vi "Pot Single Line-UR6060.vi"() -> ()   [LabVIEW 2017]
uses:
  Shared Components/Config Manager Class/Type Definitions/Potting Parameters.ctl
  <vilib>/Utility/error.llb/DialogType.ctl
  Shared Components/Config Manager Class/Type Definitions/Camera Enum.ctl
  Shared Components/Gantry Class/Type Definitions/Init_Modes.ctl
  Shared Components/Gantry Class/Type Definitions/Virtual Modes.ctl
  Shared Components/Config Manager Class/Type Definitions/Potting Surface Type.ctl
  Shared Components/Gantry Class/Gantry Class.lvclass
  Shared Components/SyringeTool Class/SyringeTool Class.lvclass
  Shared Components/WorkTable Class/WorkTable Class.lvclass
  Shared Components/Vec3d Class/Vec3d Class.lvclass
panel:
  out "error out":errorcluster
  in  "Potting Parameters":T1={"Curing Param A"=0.0, "Curing Param B"=0.0, "Speed Nominal"=0.5, "Time Nominal"=2.0, "Turn-on Time"=0.5, "Turn-off Time"=0.1, "Safe Height Offset"=0.0, "Tip Height"=0.18, "Width of Line"=0.0, "Number of lines"=1.0, "Distance between lines"=0.1}
  out "Image":T2(plugin-control)
  in  "stop":bool
  in  "Config Folder":path=path "C:/Users/Husker/Desktop/gantry/Config"
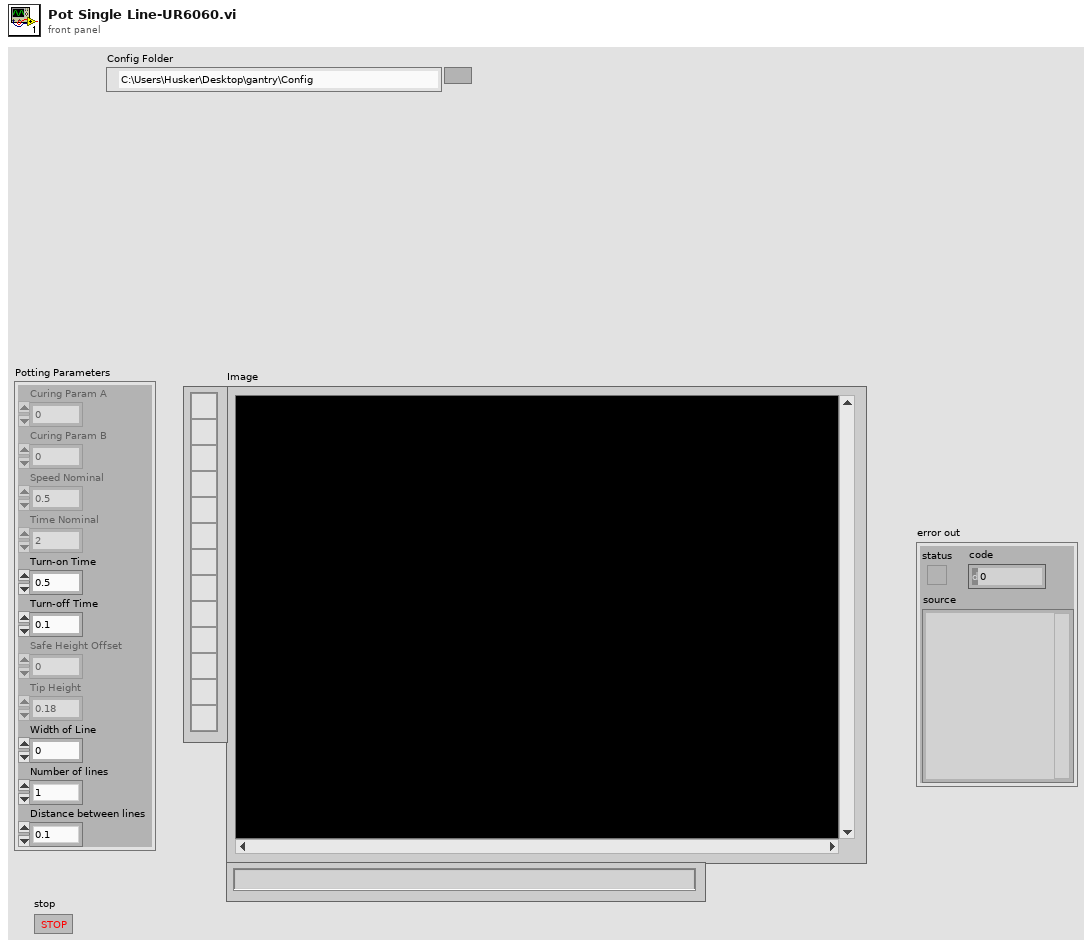
[diagram p1: front panel]
types:
  T1 = typedef "Potting Parameters.ctl" = cluster{"Curing Param A":dbl, "Curing Param B":dbl, "Speed Nominal":dbl, "Time Nominal":dbl, "Turn-on Time":dbl, "Turn-off Time":dbl, "Safe Height Offset":dbl, "Tip Height":dbl, "Width of Line":dbl, "Number of lines":dbl, "Distance between lines":dbl}
  T2 = typedef "IMAQ Image.ctl" = refnum<image>
  T3 = typedef "Virtual Modes.ctl" = enum16{"Nonvirtual", "Pseudovirtual", "Virtual"}
  T4 = typedef "Init_Modes.ctl" = enum16{"Full", "Robot Only", "Dispenser Only", "Cameras Only", "Robot and Cameras", "Robot and Cameras and Dispenser", "Manifold Only"}
  T5 = typedef "Camera Enum.ctl" = enum16{"GANTRY HEAD", "NEEDLE CALIBRATION X", "NEEDLE CALIBRATION Y", "STAND CAMERA", "SIMRAN WEBCAM"}
  T6 = typedef "DialogType.ctl" = u16
  T7 = typedef "Worktable_Syringe.ctl" = cluster{"Syringe Holder":enum16{"Empty", "Populated", "Calibrated"}, "Mixing Time":timestamp, "Tip Offset":refnum<class "Vec3d Class.lvclass">}
  T8 = typedef "Potting Surface Type.ctl" = enum16{"default", "hdi_edge_pads", "bbm_edge_pads", "address_pads"}
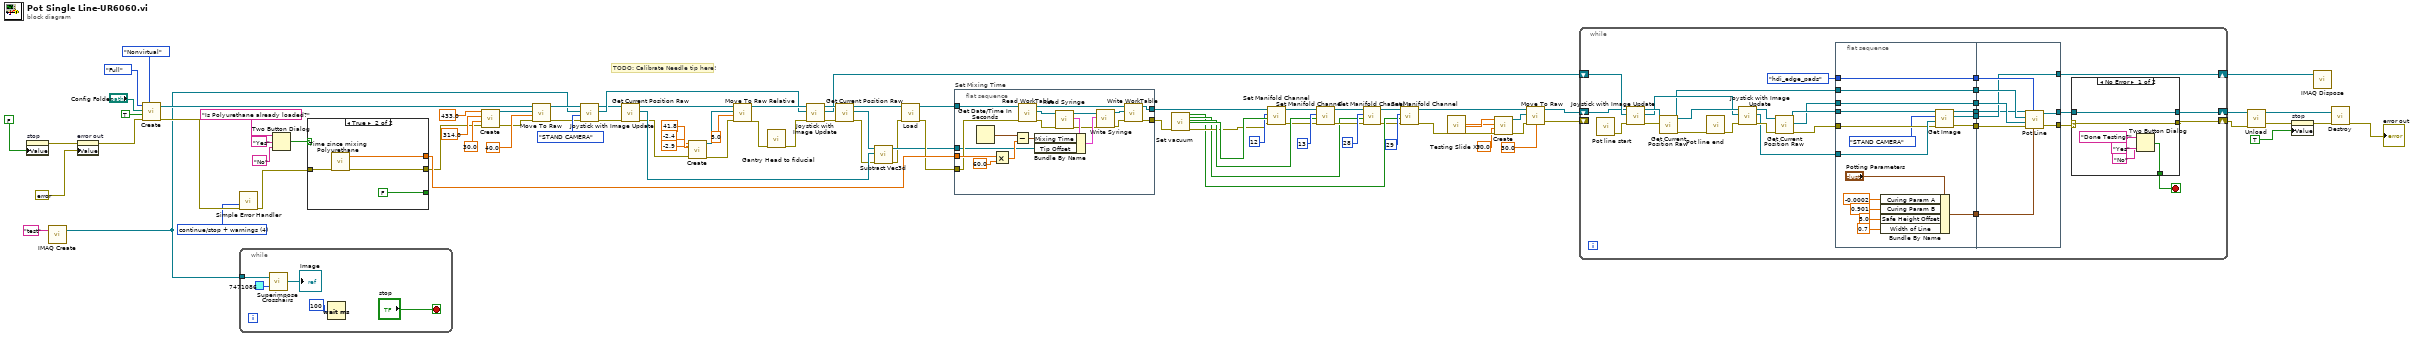
[diagram p0: block diagram]
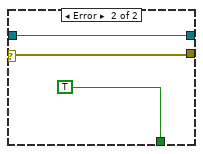
[diagram p2: hidden frame]
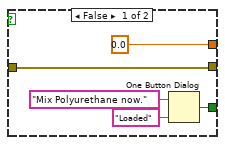
[diagram p3: hidden frame]
diagram:
  w79 = T6 4 items=["no dialog", "OK message", "continue or stop message", "OK message + warnings", "continue/stop + warnings"] ("type of dialog (OK msg:1)")
  # "TODO: Calibrate Needle tip here!"
  n1 = property on="stop" class="Bool (strict)"("Value"=FALSE) -> (error out=w23:errorcluster)  [unwired: 2 in, 1 out]
  n2 = call "IMAQ Create"("Image Name"="test") -> ("New Image"=w48:T2)  [unwired: 4 in, 1 out]
  n3 = property on="error out" class="Clust (strict)"(error in=w23, "Value"=errorcluster {"status"=FALSE, "code"=0, "source"=""} ("error in (no error)")) -> (error out=w20:errorcluster)  [unwired: 1 in, 1 out]
  n4 = call "Create.vi"("Virtual Mode"=Virtual_Modes."Nonvirtual", "error in"=w20, "HOME?"=TRUE, "Config Folder"="Config Folder", "Init Mode"=Init_Modes."Full") -> ("error out"=w81:errorcluster, "Gantry out"=w72:refnum<class "Gantry Class.lvclass">)  [unwired: 5 in]
  n5 = call <vilib>:"Simple Error Handler.vi"("type of dialog (OK msg:1)"=w79, "error in (no error)"=w81) -> ("error out"=w80:errorcluster)  [unwired: 3 in, 4 out]
  n6 = while {
    tunnel: w48 -> [w93]
    stop <- "stop" stop-if-true
    n7 = call "Superimpose Crosshairs.vi"("Grid Line Color"=u32 7471086, "Refnum in"=w93) -> ("Refnum out"=→"Image":T2)
    n8 = Wait (ms)(milliseconds to wait=u32 100) -> ()  [unwired: 1 out]
  }
  n9 = Two Button Dialog(message="Is Polyurethane already loaded?", 1:"No" ("F button name (\"Cancel\")"), 2:"Yes" ("T button name (\"OK\")")) -> (T button?=w85:bool)
  n10 = case shown="True" w85 {
    tunnel: w80 -> [w96 w103]
    tunnel: [w96 w102] -> w71
    tunnel: [0.0 ("minutes") w104] -> w89
    tunnel: [w97 FALSE ("true")] -> _
    frame False {
      n11 = One Button Dialog(message="Mix Polyurethane now.", button name ("OK")="Loaded") -> (true=w97:bool)
    }
    frame True {
      n12 = call "Time since mixing Polyurethane"("error in (no error)"=w103) -> ("minutes"=w104:dbl, "error out"=w102:errorcluster)  [unwired: 16 in, 1 out]
    }
  }
  n13 = call "Create.vi"("error in"=w71, "Z"=30.0, "Y"=314.0, "X"=433.0) -> ("error out"=w76:errorcluster, "Vec3d Class out"=w78:refnum<class "Vec3d Class.lvclass">)  [unwired: 6 in]
  n14 = call-dynamic "Move To Raw.vi"("error in"=w76, "Speed"=40.0, "Destination"=w78, "Gantry in"=w72) -> ("error out"=w50:errorcluster, "Gantry out"=w51:refnum<class "Gantry Class.lvclass">)  [unwired: 6 in]
  n15 = call-dynamic "Joystick with Image Update.vi"("error in (no error)"=w50, "Camera Name"=Camera_Enum."STAND CAMERA", "Image In"=w48, "Gantry Class in"=w51) -> ("error out"=w56:errorcluster, "Image Out"=w59:T2, "Gantry Class out"=w57:refnum<class "Gantry Class.lvclass">)  [unwired: 5 in]
  n16 = call-dynamic "Get Current Position Raw.vi"("error in"=w56, "Gantry in"=w57) -> ("error out"=w53:errorcluster, "Vec3d Class out"=w54:refnum<class "Vec3d Class.lvclass">, "Gantry out"=w55:refnum<class "Gantry Class.lvclass">)  [unwired: 7 in]
  n17 = call "Create.vi"("error in"=w53, "Z"=-2.9, "Y"=-2.4, "X"=41.8) -> ("error out"=w58:errorcluster, "Vec3d Class out"=w63:refnum<class "Vec3d Class.lvclass">)  [unwired: 6 in]
  n18 = call-dynamic "Move To Raw Relative.vi"("error in"=w58, "Speed(mm/s)"=5.0 ("Speed"), "Delta"=w63, "Gantry in"=w55) -> ("error out"=w60:errorcluster, "Gantry out"=w61:refnum<class "Gantry Class.lvclass">)  [unwired: 6 in]
  n19 = call "Gantry Head to fiducial"("error in (no error)"=w60) -> ("error out"=w67:errorcluster)  [unwired: 9 in, 1 out]
  n20 = call-dynamic "Joystick with Image Update.vi"("error in (no error)"=w67, "Image In"=w59, "Gantry Class in"=w61) -> ("error out"=w69:errorcluster, "Image Out"=w40:T2, "Gantry Class out"=w70:refnum<class "Gantry Class.lvclass">)  [unwired: 6 in]
  n21 = call-dynamic "Get Current Position Raw.vi"("error in"=w69, "Gantry in"=w70) -> ("error out"=w45:errorcluster, "Vec3d Class out"=w68:refnum<class "Vec3d Class.lvclass">, "Gantry out"=w47:refnum<class "Gantry Class.lvclass">)  [unwired: 7 in]
  n22 = call "Subtract Vec3d.vi"("error in (no error)"=w45, "Vec3d in 2"=w54, "Vec3d in 1"=w68) -> ("error out"=w44:errorcluster, "Vec3d Class out"=w46:refnum<class "Vec3d Class.lvclass">)  [unwired: 7 in]
  n23 = call "Load.vi"("error in"=w44, "Gantry in"=w47) -> ("error out"=w83:errorcluster, "SyringeTool out"=w84:refnum<class "SyringeTool Class.lvclass">)  [unwired: 8 in]
  n24 = flat-sequence "Set Mixing Time" {
    tunnel: w84 -> [w119]
    tunnel: w89 -> [w123]
    tunnel: w83 -> [w118]
    tunnel: [w107] -> w4
    tunnel: [w106] -> w3
    tunnel: w46 -> [w105]
    frame #0 {
      n25 = Get Date/Time In Seconds() -> (seconds since 1Jan1904=w121:timestamp)
      n26 = Multiply(x=w123, y=60.0) -> (x*y=w120:dbl)
      n27 = Subtract(x=w121, y=w120) -> (x-y=w115:timestamp)
      n28 = call-dynamic "Read WorkTable.vi"("error in"=w118, "Gantry Class in"=w119) -> ("error out"=w110:errorcluster, "WorkTable Class.lvclass"=w117:refnum<class "WorkTable Class.lvclass">, "Gantry Class out"=w112:refnum<class "SyringeTool Class.lvclass">)  [unwired: 7 in]
      n29 = call "Read Syringe.vi"("error in"=w110, "WorkTable in"=w117) -> ("error out"=w109:errorcluster, "Syringe"=w116:T7, "WorkTable out"=w113:refnum<class "WorkTable Class.lvclass">)  [unwired: 7 in]
      n30 = Bundle By Name(cluster=w116, "Mixing Time"=w115, "Tip Offset"=w105) -> (w114:T7)
      n31 = call-dynamic "Write Syringe.vi"("error in (no error)"=w109, "Syringe"=w114, "WorkTable Class in"=w113) -> ("error out"=w108:errorcluster, "WorkTable Class out"=w111:refnum<class "WorkTable Class.lvclass">)  [unwired: 7 in]
      n32 = call-dynamic "Write WorkTable.vi"("error in (no error)"=w108, "WorkTable Class.lvclass"=w111, "Gantry Class in"=w112) -> ("error out"=w106:errorcluster, "Gantry Class out"=w107:refnum<class "SyringeTool Class.lvclass">)  [unwired: 7 in]
    }
  }
  n33 = call "Set vacuum"("error in (no error)"=w3) -> ("Vacuum 2B"=w6:bool, "Vacuum 2A"=w8:bool, "Vacuum 1B"=w13:bool, "Vacuum 1A"=w19:bool, "error out"=w12:errorcluster)  [unwired: 13 in, 1 out]
  n34 = call-dynamic "Set Manifold Channel.vi"("error in"=w12, "On/Off"=w19, "Manifold Channel"=12, "Gantry in"=w4) -> ("error out"=w11:errorcluster, "Gantry out"=w14:refnum<class "SyringeTool Class.lvclass">)  [unwired: 6 in]
  n35 = call-dynamic "Set Manifold Channel.vi"("error in"=w11, "On/Off"=w13, "Manifold Channel"=13, "Gantry in"=w14) -> ("error out"=w10:errorcluster, "Gantry out"=w9:refnum<class "SyringeTool Class.lvclass">)  [unwired: 6 in]
  n36 = call-dynamic "Set Manifold Channel.vi"("error in"=w10, "On/Off"=w8, "Manifold Channel"=28, "Gantry in"=w9) -> ("error out"=w5:errorcluster, "Gantry out"=w7:refnum<class "SyringeTool Class.lvclass">)  [unwired: 6 in]
  n37 = call-dynamic "Set Manifold Channel.vi"("error in"=w5, "On/Off"=w6, "Manifold Channel"=29, "Gantry in"=w7) -> ("error out"=w2:errorcluster, "Gantry out"=w1:refnum<class "SyringeTool Class.lvclass">)  [unwired: 6 in]
  n38 = call "Testing Slide XY"("error in (no error)"=w2) -> ("Y"=w38:dbl, "X"=w39:dbl, "error out"=w34:errorcluster)  [unwired: 15 in, 1 out]
  n39 = call "Create.vi"("error in"=w34, "Z"=30.0, "Y"=w38, "X"=w39) -> ("error out"=w35:errorcluster, "Vec3d Class out"=w37:refnum<class "Vec3d Class.lvclass">)  [unwired: 6 in]
  n40 = call-dynamic "Move To Raw.vi"("error in"=w35, "Speed"=30.0, "Destination"=w37, "Gantry in"=w1) -> ("error out"=w41:errorcluster, "Gantry out"=w32:refnum<class "SyringeTool Class.lvclass">)  [unwired: 6 in]
  n41 = while {
    shift-right: [w130] -> w42
    shift-left: w40 -> [w148]
    shift-right: [w124] -> w30
    shift-left: w41 -> [_]
    shift-right: [w125] -> w31
    shift-left: w32 -> [w128]
    stop <- w138 stop-if-true
    n42 = call "Pot line start"() -> ("error out"=w141:errorcluster)  [unwired: 10 in, 1 out]
    n43 = call-dynamic "Joystick with Image Update.vi"("error in (no error)"=w141, "Image In"=w148, "Gantry Class in"=w128) -> ("error out"=w142:errorcluster, "Image Out"=w151:T2, "Gantry Class out"=w153:refnum<class "SyringeTool Class.lvclass">)  [unwired: 6 in]
    n44 = call-dynamic "Get Current Position Raw.vi"("error in"=w142, "Gantry in"=w153) -> ("error out"=w140:errorcluster, "Vec3d Class out"=w146:refnum<class "Vec3d Class.lvclass">, "Gantry out"=w152:refnum<class "SyringeTool Class.lvclass">)  [unwired: 7 in]
    n45 = call "Pot line end"("error in (no error)"=w140) -> ("error out"=w139:errorcluster)  [unwired: 9 in, 1 out]
    n46 = call-dynamic "Joystick with Image Update.vi"("error in (no error)"=w139, "Image In"=w151, "Gantry Class in"=w152) -> ("error out"=w149:errorcluster, "Image Out"=w132:T2, "Gantry Class out"=w150:refnum<class "SyringeTool Class.lvclass">)  [unwired: 6 in]
    n47 = call-dynamic "Get Current Position Raw.vi"("error in"=w149, "Gantry in"=w150) -> ("error out"=w143:errorcluster, "Vec3d Class out"=w145:refnum<class "Vec3d Class.lvclass">, "Gantry out"=w147:refnum<class "SyringeTool Class.lvclass">)  [unwired: 7 in]
    n48 = flat-sequence {
      tunnel: w143 -> [w158]
      tunnel: Potting_Surface_Type."hdi_edge_pads" ("Potting Surface Type") -> [w167]
      tunnel: w145 -> [w168]
      tunnel: w146 -> [w169]
      tunnel: w147 -> [w159]
      tunnel: [w169] -> w137
      tunnel: [w168] -> w136
      tunnel: [w167] -> w135
      tunnel: [w157] -> w134
      tunnel: [w165] -> w133
      tunnel: w132 -> [w160]
      tunnel: [w155] -> w131
      tunnel: [w154] -> w129
      tunnel: w137 -> [w178]
      tunnel: w136 -> [w177]
      tunnel: w135 -> [w176]
      tunnel: w134 -> [w175]
      tunnel: w133 -> [w174]
      tunnel: [w173] -> w130
      tunnel: w131 -> [w173]
      tunnel: w129 -> [w172]
      tunnel: [w171] -> w127
      tunnel: [w170] -> w126
      frame #0 {
        n49 = Bundle By Name(cluster="Potting Parameters", "Curing Param A"=-0.0002, "Curing Param B"=0.901, "Safe Height Offset"=5.0, "Width of Line"=0.7 ("Pot Length Scale")) -> (w165:T1)
        n50 = call-dynamic "Get Image.vi"("error in"=w158, "Image In"=w160, "Camera Name"=Camera_Enum."STAND CAMERA", "Gantry in"=w159) -> ("error out"=w157:errorcluster, "Image Out"=w155:T2, "Gantry out"=w154:refnum<class "SyringeTool Class.lvclass">)  [unwired: 4 in, 1 out]
      }
      frame #1 {
        n51 = call-dynamic "Pot Line.vi"("Potting Parameters"=w174, "Potting Surface Type"=w176, "error in"=w175, "End Position"=w177, "Start Position"=w178, "SyringeTool in"=w172) -> ("error out"=w170:errorcluster, "SyringeTool out"=w171:refnum<class "SyringeTool Class.lvclass">)  [unwired: 4 in]
      }
    }
    n52 = case shown="No Error" w126 {
      selector: w126 -> [w180 w187]
      tunnel: [w180 w187] -> w124
      tunnel: [w181 TRUE ("Done Testing?")] -> w138
      tunnel: w127 -> [w179 w185]
      tunnel: [w179 w185] -> w125
      frame No Error {
        n53 = Two Button Dialog(message="Done Testing?", 1:"No" ("F button name (\"Cancel\")"), 2:"Yes" ("T button name (\"OK\")")) -> (T button?=w181:bool)
      }
      frame Error {
      }
    }
  }
  n54 = call "Unload.vi"("error in"=w30, "SyringeTool in"=w31) -> ("error out"=w25:errorcluster, "Gantry out"=w29:refnum<class "Gantry Class.lvclass">)  [unwired: 8 in]
  n55 = property on="stop" class="Bool (strict)"(error in=w25, "Value"=TRUE ("stop")) -> (error out=w24:errorcluster)  [unwired: 1 in, 1 out]
  n56 = call "IMAQ Dispose"("Image"=w42) -> ()  [unwired: 5 in, 1 out]
  n57 = call "Destroy.vi"("error in"=w24, "Gantry Class in"=w29) -> ("error out"=→"error out":errorcluster)  [unwired: 9 in]
